vi "battery.vi"(11 "MS":dbl[](array[numeric])) -> (0 "Current Usage":dbl, 1 "Percentage":dbl, 2 "Present Voltage":dbl, 3 "Present Current":dbl)   [LabVIEW 2015]
uses:
  <vilib>/imath/engines/lvmath2/RunTimeEngine/NodeEndStatement/NIMS_NodeEndStatement_Output.vi
  <instcachedir>/0/NIMS_NodeEndStatement_Output_53EC0D466D134D7ABD903AC30B43404B.lvgen/NIMS_NodeEndStatement_Output_53EC0D466D134D7ABD903AC30B43404B_001.vi
  <vilib>/imath/engines/lvmath2/RunTimeEngine/ErrorHandling/NIMS_Finalize Error.vi
panel:
  in  "mc":dbl=6600.0
  in  "mv":dbl=16.8
  in  "cp":dbl=100.0
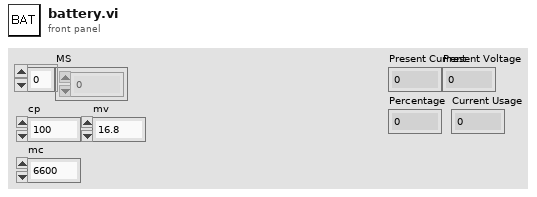
[diagram p1: front panel]
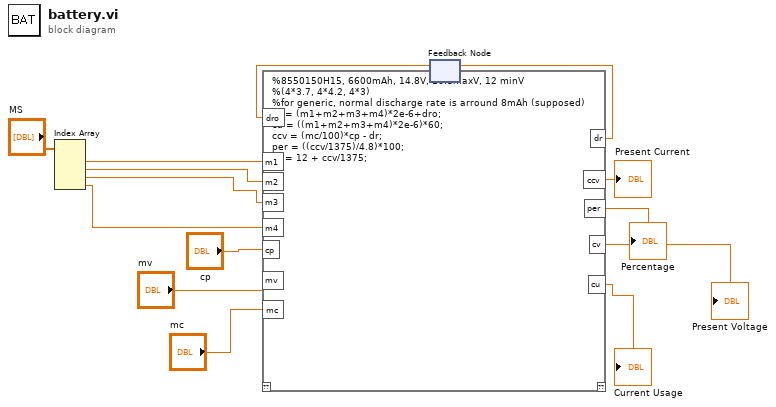
[diagram p0: block diagram]
diagram:
  n1 = Index Array ("Index Array 5")(array="MS") -> (element #1=w13:dbl, element #2=w12:dbl, element #3=w11:dbl, element #4=w10:dbl)  [unwired: 4 in]
  n2 = feedback #1() -> (w8:dbl)  [unwired: 1 in]
  n3 = mathscript code="%8550150H15, 6600mAh, 14.8V, 16.8maxV, 12 minV\n%(4*3.7, 4*4.2, 4*3)\n%for generic, normal discharge rate is arround 8mAh (supposed)\ndr = (m1+m2+m3+m4)*2e-6+dro;\ncu = ((m1+m2+m3+m4)*2e-6)*60;\nccv = (mc/100)*cp - dr;\nper = ((ccv/1375)/4.8)*100;\ncv = 12 + ccv/1375;"("m1"=w13, "m2"=w12, "m3"=w11, "m4"=w10, "cp"="cp", "dro"=w8, "mv"="mv", "mc"="mc") -> ("dr"=w1:dbl, "ccv"=→"Present Current":dbl, "per"=→"Percentage":dbl, "cv"=→"Present Voltage":dbl, "cu"=→"Current Usage":dbl)  [unwired: 1 in, 1 out]
  n4 = feedback-in #1(w1) -> ()
